vi "Btn2.vi"(8 "error in (no error)":errorcluster, 11 "Machine d'état in":refnum<class "Machine d'état.lvclass">) -> (0 "error out":errorcluster, 3 "Machine d'état out":refnum<class "Machine d'état.lvclass">)   [LabVIEW 2020, in "Machine d'état.lvlib" / "Machine d'état.lvclass"]
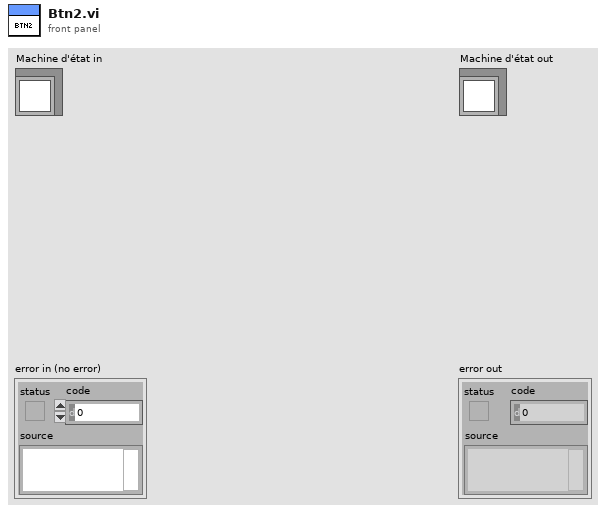
[diagram p1: front panel]
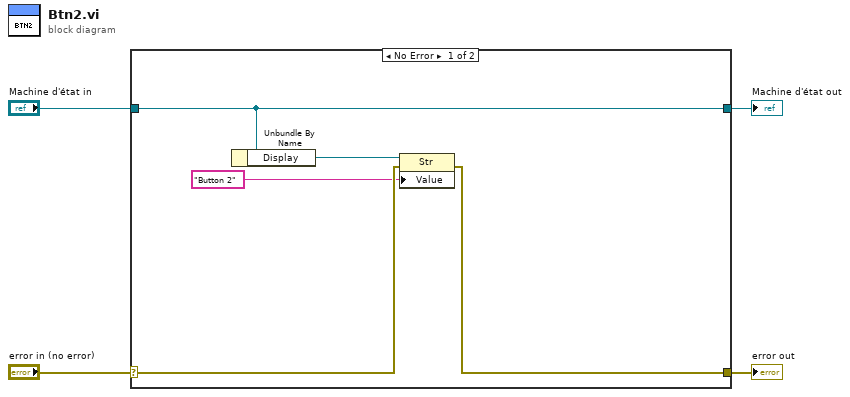
[diagram p0: block diagram]
diagram:
  n1 = case shown="No Error" "error in (no error)" {
    selector: "error in (no error)" -> [w7 w11]
    tunnel: [w6 w11] -> w3
    tunnel: [w9 w10] -> w1
    tunnel: "Machine d'état in" -> [w9 w10]
    frame No Error {
      n2 = Unbundle By Name(w9) -> ("Display"=w8:refnum<vi>)
      n3 = property class="Str"(reference=w8, error in=w7, "Value"="Button 2" ("event data")) -> (error out=w6:errorcluster)  [unwired: 1 out]
    }
    frame Error {
    }
  }
  "error out" <- w3
  "Machine d'état out" <- w1
